vi "BRig_RT__Case_Exp__State_initTrial2__Laser_Reward.vi"(1 "input_L_OnOff":u16, 2 "input_L_Block":u16, 3 "input_L_Trial":u16, 4 "input_L_Probability":u16, 8 "input_iSpout":u16, 10 "input_sState_start":u16, 12 "input_LaserSwitch":bool) -> (16 "output_LR_Event":bool, 17 "output_LR_Event_num":u16, 18 "output_LR_Laser":bool, 19 "output_LR_Laser_num":u16)   [LabVIEW 2014]
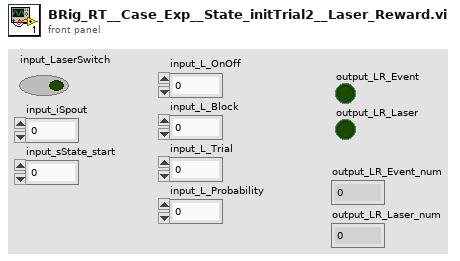
[diagram p1: front panel]
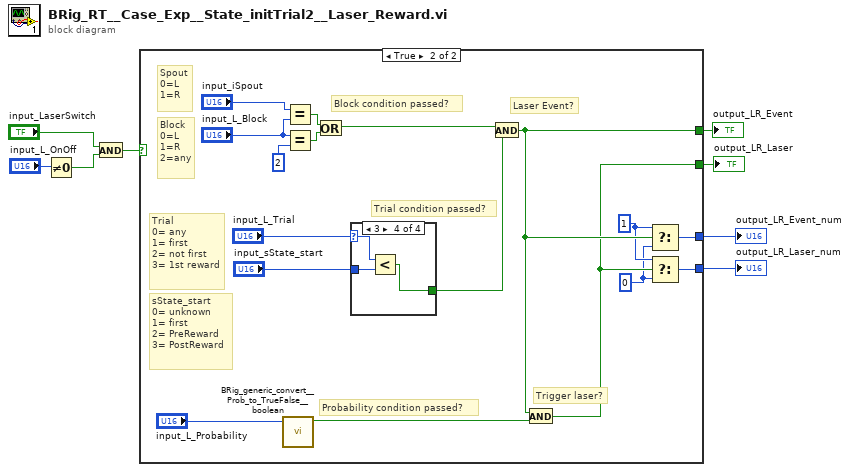
[diagram p0: block diagram]
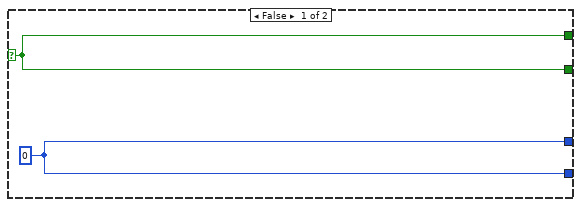
[diagram p2: hidden frame]
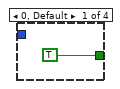
[diagram p3: hidden frame]
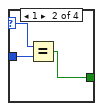
[diagram p4: hidden frame]
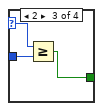
[diagram p5: hidden frame]
diagram:
  n1 = Not Equal To 0?(x="input_L_OnOff") -> (x != 0?=w7:bool)
  n2 = And(x="input_LaserSwitch", y=w7) -> (x .and. y?=w5:bool)
  n3 = case shown="True" w5 {
    selector: w5 -> [w10 _]
    tunnel: [w10 w16] -> w4
    tunnel: [w10 w15] -> w3
    tunnel: [w9 w12] -> w2
    tunnel: [w9 w11] -> w1
    frame False {
      w9 = u16 0 ("y")
    }
    frame True {
      w13 = u16 0 ("y")
      w14 = u16 1 ("y")
      # "Trigger laser?"
      # "Laser Event?"
      # "Trial condition passed?"
      # "sState_start\n0= unknown\n1= first\n2= PreReward\n3= PostReward"
      # "Probability condition passed?"
      # "Trial\n0= any\n1= first\n2= not first\n3= 1st reward"
      # "Block condition passed?"
      # "Spout\n0=L\n1=R"
      # "Block\n0=L\n1=R\n2=any"
      n4 = call "BRig_generic_convert__Prob_to_TrueFalse__boolean.vi"("input_probability_u16"="input_L_Probability") -> ("output_TF"=w17:bool)  [unwired: 10 in]
      n5 = Equal?(x="input_iSpout", y="input_L_Block") -> (x = y?=w27:bool)
      n6 = Equal?(x="input_L_Block", y=u16 2) -> (x = y?=w26:bool)
      n7 = Or(x=w27, y=w26) -> (x .or. y?=w19:bool)
      n8 = case shown="3" "input_L_Trial" {
        selector: "input_L_Trial" -> [_ w30 w33 w36]
        tunnel: [TRUE w29 w32 w35] -> w18
        tunnel: "input_sState_start" -> [_ w31 w34 w37]
        frame 0, Default {
        }
        frame 1 {
          n9 = Equal?(x=w30, y=w31) -> (x = y?=w29:bool)
        }
        frame 2 {
          n10 = Greater Or Equal?(x=w33, y=w34) -> (x >= y?=w32:bool)
        }
        frame 3 {
          n11 = Less?(x=w36, y=w37) -> (x < y?=w35:bool)
        }
      }
      n12 = And(x=w19, y=w18) -> (x .and. y?=w16:bool)
      n13 = And(x=w16, y=w17) -> (x .and. y?=w15:bool)
      n14 = Select(t=w14, s=w16, f=w13) -> (s? t:f=w12:u16)
      n15 = Select(t=w14, s=w15, f=w13) -> (s? t:f=w11:u16)
    }
  }
  "output_LR_Event" <- w4
  "output_LR_Laser" <- w3
  "output_LR_Event_num" <- w2
  "output_LR_Laser_num" <- w1
